vi "modified Sort Scan Parameters.vi"(8 "error in (no error)":errorcluster, 11 "data":T1 {"Scan parameters"."Rate" format="%.2f"; "Scan parameters"."Step" format="%#_6p"; "Scan parameters"."End" format="%#_6p"; "Scan parameters"."Start" format="%#_6p"}) -> (0 "error out":errorcluster, 1 "Sorted scan parameters":cluster{T6}[](array[cluster])=[{[{"Start"=0.14, "End"=-0.060000000000000005, "Step"=-0.060000000000000005, "Rate"=0.0, "wait (ms)"=10000, "Address"="Dev2/ao0", "channel"=1}]}, {[{"Start"=0.14, "End"=-0.060000000000000005, "Step"=-0.060000000000000005, "Rate"=0.0, "wait (ms)"=10000, "Address"="Dev2/ao0", "channel"=1}]}, {[{"Start"=0.14, "End"=-0.060000000000000005, "Step"=-0.060000000000000005, "Rate"=0.0, "wait (ms)"=10000, "Address"="Dev2/ao0", "channel"=1}, {"Start"=0.14, "End"=-0.060000000000000005, "Step"=-0.060000000000000005, "Rate"=0.0, "wait (ms)"=10000, "Address"="Dev2/ao0", "channel"=1}]}] {"?"."Rate" format="%.2f"; "?"."Step" format="%#_6p"; "?"."End" format="%#_6p"; "?"."Start" format="%#_6p"}, 2 "Sorted scan control":cluster{T2}[](array[cluster])=[{[{"Priority"=enum."Priority 0", "Scan name"=enum."DSA_Vsg2"}]}, {[{"Priority"=enum."Priority 1", "Scan name"=enum."DSA_Vamp"}]}, {[{"Priority"=enum."Priority 2", "Scan name"=enum."DSA_Vsg1"}, {"Priority"=enum."Priority 2", "Scan name"=enum."DSA_Vsg3"}]}])   [LabVIEW 2016]
uses:
  <userlib>/LevyLab/Transport/SweepControl/Typedefs/ScanControl.ctl
  <userlib>/LevyLab/Transport/SweepControl/Typedefs/Cluster - ScanControl.ctl
  <userlib>/LevyLab/Transport/SweepControl/Typedefs/Enum - Priority.ctl
  <userlib>/LevyLab/Transport/SweepControl/Typedefs/Enum - Action.ctl
  <userlib>/LevyLab/Transport/SweepControl/Typedefs/ScanParamters.ctl
  <userlib>/LevyLab/Transport/SweepControl/Typedefs/Cluster - ScanParamters.ctl
  <userlib>/LevyLab/Transport/SweepControl/Typedefs/Sweep Control Configuration--Cluster.ctl
  <userlib>/LevyLab/Transport/SweepControl/Typedefs/Enum - Experiments.ctl
  <userlib>/LevyLab/Transport/SweepControl/SweepControl.lvclass
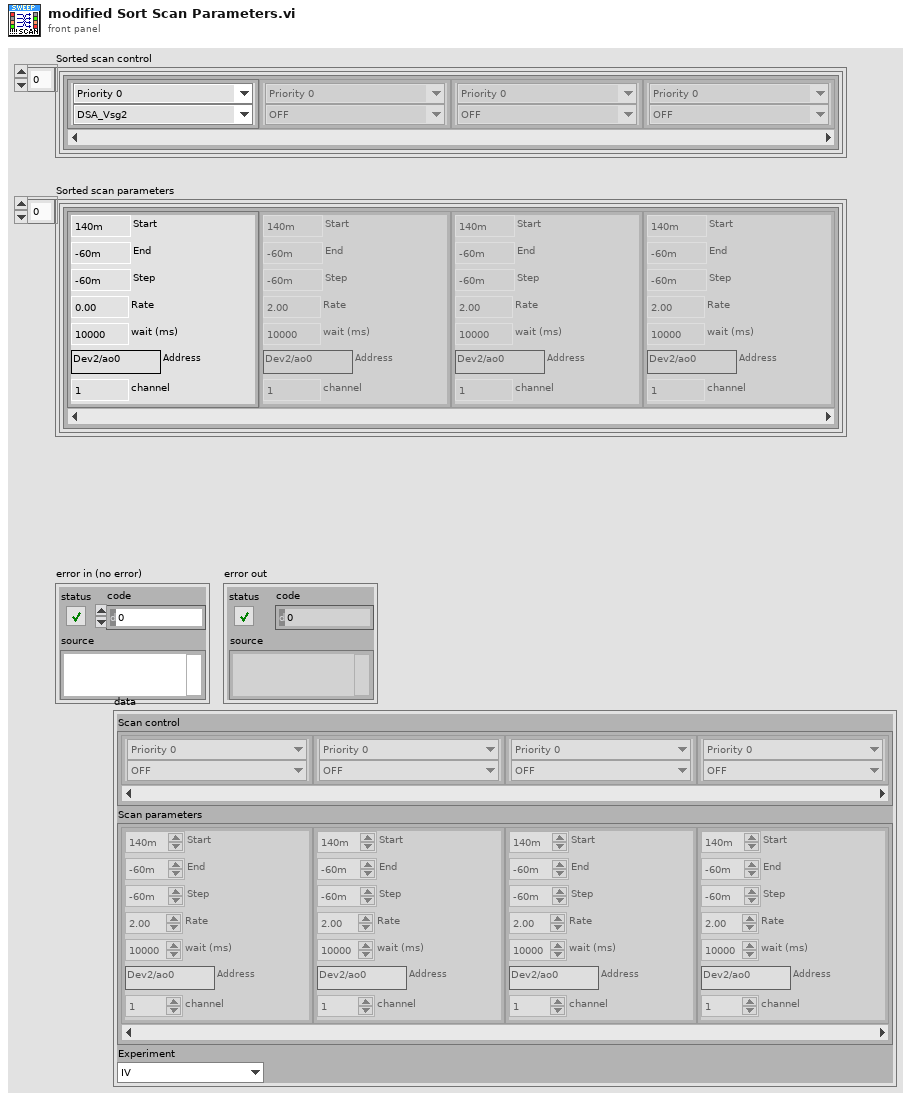
[diagram p1: front panel]
types:
  T1 = typedef "SweepControl.lvclass/Sweep Control Configuration--Cluster.ctl" = cluster{"Scan control":T2, "Scan parameters":T6, "Experiment":T8}
  T2 = typedef "SweepControl.lvclass/ScanControl.ctl" = T3[]
  T3 = typedef "SweepControl.lvclass/Cluster - ScanControl.ctl" = cluster{"Priority":T4, "Scan name":T5}
  T4 = typedef "SweepControl.lvclass/Enum - Priority.ctl" = enum16{"Priority 0", "Priority 1", "Priority 2", "Priority 3", "Priority 4", "Priority 5"}
  T5 = typedef "SweepControl.lvclass/Enum - Action.ctl" = enum16{"OFF", "DSA_Vamp", "DSA_freq", "DSA_Vsg1", "DSA_Vsg2", "DSA_Vsg3", "DAQ_Vbg", "B_Field", "Humidity", "Temp", "MW_freq1", "MW_freq2", "MW_amplitude1", "MW_amplitude2"}
  T6 = typedef "SweepControl.lvclass/ScanParamters.ctl" = T7[]
  T7 = typedef "SweepControl.lvclass/Cluster - ScanParamters.ctl" = cluster{"Start":dbl, "End":dbl, "Step":dbl, "Rate":dbl, "wait (ms)":u32, "Address":string, "channel":i32}
  T8 = typedef "SweepControl.lvclass/Enum - Experiments.ctl" = enum16{"IV", "Lockin_time", "Lockin_Vsg", "Lockin (experimental)", "Lockin_Vsg_JKISM"}
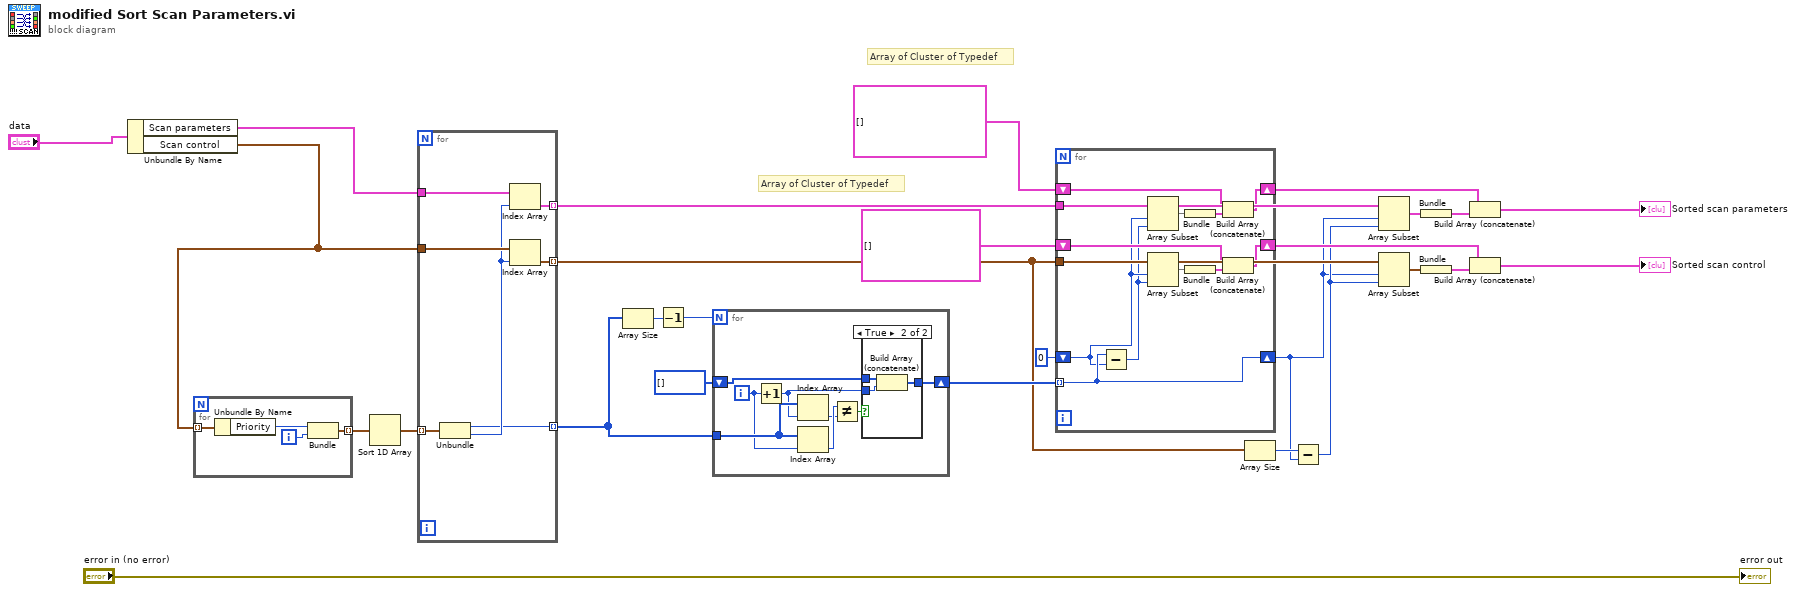
[diagram p0: block diagram]
diagram:
  # "Array of Cluster of Typedef"
  # "Array of Cluster of Typedef"
  n1 = Unbundle By Name("data") -> ("Scan parameters"=w6:T6, "Scan control"=w5:T2)
  n2 = for {
    tunnel: w5 -> [w28] mode=indexing
    tunnel: [w31] -> w27 mode=indexing
    i -> [w29]
    n3 = Unbundle By Name(w28) -> ("Priority"=w30:T4)
    n4 = Bundle("Priority"=w30, w29) -> (w31:cluster{"Priority":T4, i32})  [unwired: 1 in]
  }
  n5 = Sort 1D Array(array=w27) -> (sorted array=w26:cluster{"Priority":T4, i32}[])
  n6 = for {
    tunnel: w26 -> [w38] mode=indexing
    tunnel: w5 -> [w37]
    tunnel: [w36] -> w16 mode=indexing
    tunnel: w6 -> [w35]
    tunnel: [w34] -> w12 mode=indexing
    tunnel: [w32] -> w23 mode=indexing
    n7 = Unbundle(w38) -> ("Priority"=w32:T4, w33:i32)
    n8 = Index Array(array=w35, index=w33) -> (element=w34:T7)
    n9 = Index Array(array=w37, index=w33) -> (element=w36:T3)
  }
  n10 = Array Size(array=w23) -> (size(s)=w25:i32)
  n11 = Decrement(x=w25) -> (x-1=w24:i32)
  n12 = for {
    N: w24 -> [_]
    tunnel: w23 -> [w46]
    shift-right: [w42] -> w20
    shift-left: i32[] [] -> [w41]
    i -> [w39]
    n13 = Increment(x=w39) -> (x+1=w40:i32)
    n14 = Index Array(array=w46, index=w40) -> (element=w43:T4)
    n15 = Index Array(array=w46, index=w39) -> (element=w45:T4)
    n16 = Not Equal?(x=w45, y=w43) -> (x != y?=w44:bool)
    n17 = case shown="True" w44 {
      tunnel: [w47 w50] -> w42
      tunnel: w41 -> [w47 w49]
      tunnel: w40 -> [_ w48]
      frame False {
      }
      frame True {
        n18 = Build Array (concatenate)(w49, w48) -> (w50:i32[])
      }
    }
  }
  n19 = for {
    tunnel: w20 -> [w58] mode=indexing
    shift-right: [w63] -> w19
    shift-left: cluster{"Scan control":T2}[] [] -> [w62]
    tunnel: w16 -> [w61]
    shift-right: [w58] -> w10
    shift-left: 0 -> [w56]
    tunnel: w12 -> [w57]
    shift-right: [w53] -> w7
    shift-left: cluster{"Scan parameters":T6}[] [] -> [w52]
    n20 = Subtract(x=w58, y=w56) -> (x-y=w55:i32)
    n21 = Array Subset(array=w57, index=w56, length=w55) -> (w54:T7[])
    n22 = Array Subset(array=w61, index=w56, length=w55) -> (w60:T3[])
    n23 = Bundle(w54) -> (w51:cluster{T7[]})  [unwired: 1 in]
    n24 = Bundle(w60) -> (w59:cluster{T3[]})  [unwired: 1 in]
    n25 = Build Array (concatenate)(w52, w51) -> (w53:cluster{"Scan parameters":T6}[])
    n26 = Build Array (concatenate)(w62, w59) -> (w63:cluster{"Scan control":T2}[])
  }
  n27 = Array Size(array=w16) -> (size(s)=w17:i32)
  n28 = Subtract(x=w17, y=w10) -> (x-y=w11:i32)
  n29 = Array Subset(array=w12, index=w10, length=w11) -> (w13:T7[])
  n30 = Array Subset(array=w16, index=w10, length=w11) -> (w15:T3[])
  n31 = Bundle(w13) -> (w9:cluster{T7[]})  [unwired: 1 in]
  n32 = Bundle(w15) -> (w14:cluster{T3[]})  [unwired: 1 in]
  n33 = Build Array (concatenate)(w7, w9) -> (→"Sorted scan parameters":cluster{"Scan parameters":T6}[])
  n34 = Build Array (concatenate)(w19, w14) -> (→"Sorted scan control":cluster{"Scan control":T2}[])
  "error out" <- "error in (no error)"
